vi "AnalogOutput_PanelSim_Global.vi"(0 "menu":T4=enum."get", 5 "AO Channel":T3=enum."Invalid", 9 "Value Set":dbl format="%#.4f", 11 "error in (no error)":errorcluster, 12 "JSON":string) -> (10 "Value get":T1={"type"="AO", "device"="", "name"="", "data"={"<init"=FALSE, "<voltage"=0.0}}, 15 "error out":errorcluster)   [LabVIEW 2019]
doc: "This is used to set and get the last motor output values. This is needed for simulation, since we cannot read these values from the hardware.\n\nThis software is licensed. Open the labview\\readme\\WPI Robotics Library Open Source License.txt file for more information."
uses:
  AO Update Ops.ctl
  AO proto.ctl
  AO Data proto.ctl
  <vilib>/Rock Robotics/WPI/AnalogOutput/WPI_AnalogOutputChannel.ctl
panel:
  out "All Values":T1[](array[typedef])
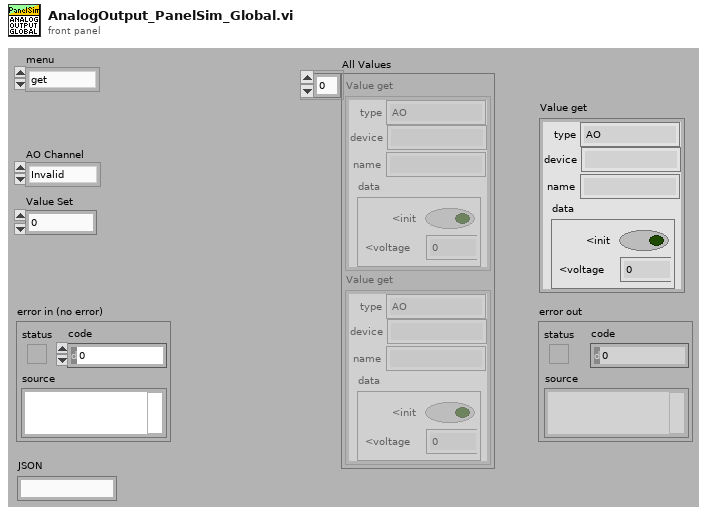
[diagram p1: front panel]
types:
  T1 = typedef "AO proto.ctl" = cluster{"type":string, "device":string, "name":string, "data":T2}
  T2 = typedef "AO Data proto.ctl" = cluster{"<init":bool, "<voltage":dbl}
  T3 = typedef "WPI_AnalogOutputChannel.ctl" = enum8{"AO MXP 0", "AO MXP 1", "Invalid"}
  T4 = typedef "AO Update Ops.ctl" = enum16{"set init", "set value", "JSON update", "set name", "transmit initial", "get", "delete", "reset"}
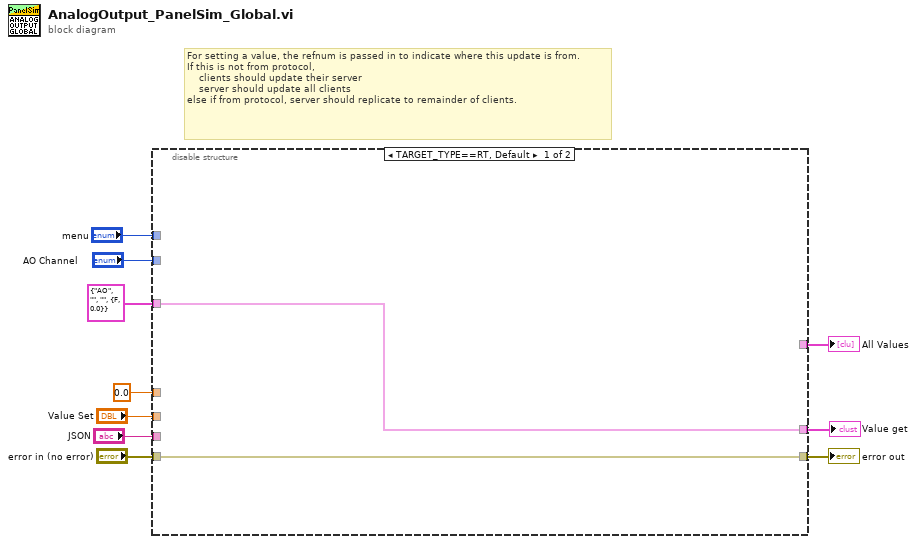
[diagram p0: block diagram]
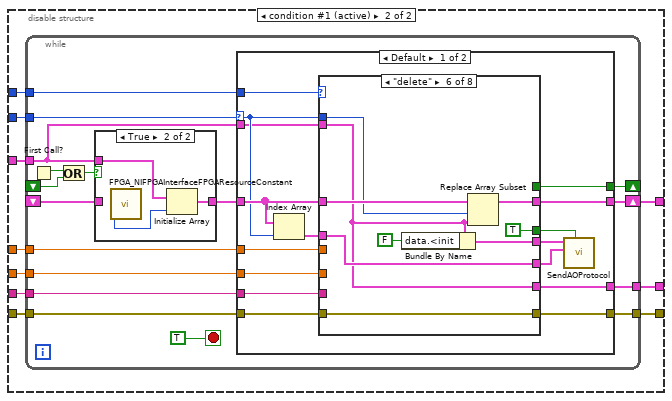
[diagram p2: hidden frame]
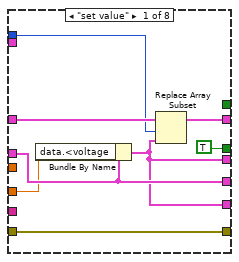
[diagram p3: hidden frame]
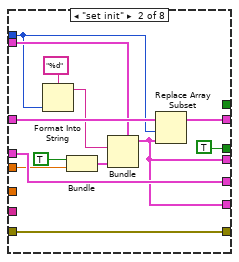
[diagram p4: hidden frame]
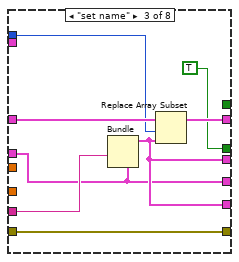
[diagram p5: hidden frame]
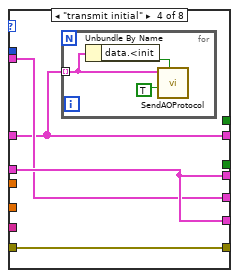
[diagram p6: hidden frame]
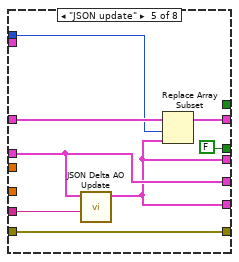
[diagram p7: hidden frame]
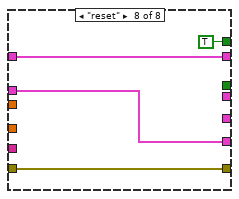
[diagram p9: hidden frame]
diagram:
  # "For setting a value, the refnum is passed in to indicate where this update is from.\nIf this is not from protocol,\n    clients should update their server\n    server should update all clients\nelse if from protocol, server should replicate to remainder of clients."
  n1 = disable-structure shown="TARGET_TYPE==RT, Default" {
    disable-tunnel: "menu" -> [_ w22]
    disable-tunnel: [w12 w21] -> w9
    disable-tunnel: "error in (no error)" -> [w12 w20]
    disable-tunnel: [_ w19] -> w7
    disable-tunnel: 0.0 ("Output") -> [_ w18]
    disable-tunnel: "Value Set" -> [_ w17]
    disable-tunnel: "AO Channel" -> [_ w16]
    disable-tunnel: [w11 w15] -> w3
    disable-tunnel: "JSON" -> [_ w14]
    disable-tunnel: T1 {"type"="AO", "device"="", "name"="", "data"={"<init"=FALSE, "<voltage"=0.0}} ("data") -> [w11 w13]
    frame condition #0 {
    }
    frame condition #1 (active) {
      n2 = while {
        tunnel: w17 -> [w39]
        tunnel: w20 -> [w35]
        shift-right: [w38] -> w19
        shift-left: _ -> [w31]
        tunnel: [w37] -> w15
        tunnel: w22 -> [w36]
        tunnel: [w34] -> w21
        tunnel: w16 -> [w29]
        tunnel: w18 -> [w30]
        tunnel: w14 -> [w28]
        tunnel: w13 -> [w27]
        shift-right: [w23] -> _
        shift-left: _ -> [w24]
        stop <- TRUE stop-if-true
        n3 = First Call?() -> (First Call?: T/F=w25:bool)
        n4 = Or(x=w25, y=w24) -> (x .or. y?=w26:bool)
        n5 = case shown="True" w26 {
          tunnel: [w119 w122] -> w32
          tunnel: w31 -> [w119 _]
          tunnel: w27 -> [_ w120]
          frame False {
          }
          frame True {
            n6 = call <vilib>:"FPGA_NIFPGAInterfaceFPGAResourceConstant.vi"() -> ("NumberOfAOChannels"=w121:u8)  [unwired: 11 out]
            n7 = Initialize Array(w120, w121) -> (w122:T1[])
          }
        }
        n8 = case shown="Default" w29 {
          selector: w29 -> [w47 _]
          tunnel: w39 -> [w55 _]
          tunnel: [w54 w118] -> w38
          tunnel: [w53 w116] -> w37
          tunnel: w36 -> [w52 _]
          tunnel: w35 -> [w51 w117]
          tunnel: [w50 w117] -> w34
          tunnel: w32 -> [w49 w118]
          tunnel: w30 -> [w48 _]
          tunnel: w28 -> [w42 _]
          tunnel: w27 -> [w41 w116]
          tunnel: [w40 _] -> w23
          frame Default {
            n9 = Index Array(array=w49, index=w47) -> (element=w46:T1)
            n10 = case shown="\"delete\"" w52 {
              tunnel: w55 -> [w57 _ _ _ _ _ _ _]
              tunnel: [w63 w76 w84 w85 w99 w107 w111 w115] -> w54
              tunnel: w49 -> [w61 w74 w82 w85 w97 w108 w111 w115]
              tunnel: [w56 w68 w79 w87 w92 w102 w109 w113] -> w53
              tunnel: [w62 w75 w83 w88 w98 w106 w110 w114] -> w50
              tunnel: w51 -> [w62 w75 w83 w88 w98 w106 w110 w114]
              tunnel: w47 -> [w59 w67 w80 _ w95 w103 _ _]
              tunnel: w48 -> [_ w64 _ _ _ _ _ _]
              tunnel: [w56 w68 w79 w87 w92 w101 _ _] -> w44
              tunnel: [w58 w72 w77 w86 w93 w104 _ _] -> w45
              tunnel: [TRUE TRUE TRUE _ FALSE TRUE _ _] -> w43
              tunnel: w46 -> [w58 w72 w77 w87 w93 w104 w109 w113]
              tunnel: w42 -> [_ _ w78 _ w94 _ _ _]
              tunnel: w41 -> [_ w71 _ w86 _ w102 _ _]
              tunnel: [_ _ _ _ _ _ _ TRUE] -> w40
              frame "set value" {
                n11 = Bundle By Name(cluster=w58, "data.<voltage"=w57) -> (w56:T1)
                n12 = Replace Array Subset(array=w61, new element=w56, index=w59) -> (w63:T1[])
              }
              frame "set init" {
                n13 = Format Into String(format string="%d", w67) -> (resulting string=w65:string)  [unwired: 2 in, 1 out]
                n14 = Bundle(TRUE, "Output"=w64) -> (w69:cluster{bool, "Output":dbl})  [unwired: 1 in]
                n15 = Bundle(cluster=w71, "device"=w65, "data"=w69) -> (w68:T1)  [unwired: 2 in]
                n16 = Replace Array Subset(array=w74, new element=w68, index=w67) -> (w76:T1[])
              }
              frame "set name" {
                n17 = Bundle(cluster=w77, "name"=w78) -> (w79:T1)  [unwired: 3 in]
                n18 = Replace Array Subset(array=w82, new element=w79, index=w80) -> (w84:T1[])
              }
              frame "transmit initial" {
                n19 = for {
                  tunnel: w85 -> [w90] mode=indexing
                  n20 = Unbundle By Name(w90) -> ("data.<init"=w89:bool)
                  n21 = call "SendAOProtocol.vi"("Send"=w89, "Initialize"=TRUE, "new"=w90) -> ()  [unwired: 9 in]
                }
              }
              frame "JSON update" {
                n22 = call "JSON Delta AO Update.vi"("Delta JSON"=w94, "input"=w93) -> ("output"=w92:T1)  [unwired: 8 in, 1 out]
                n23 = Replace Array Subset(array=w97, new element=w92, index=w95) -> (w99:T1[])
              }
              frame "delete" {
                n24 = Bundle By Name(cluster=w102, "data.<init"=FALSE) -> (w101:T1)
                n25 = Replace Array Subset(array=w108, new element=w102, index=w103) -> (w107:T1[])
              }
              frame "get" {
              }
              frame "reset" {
              }
            }
            n26 = call "SendAOProtocol.vi"("Send"=w43, "prev"=w45, "new"=w44) -> ()  [unwired: 9 in]
          }
          frame "Invalid" {
            # "Do nothing if \nchannel is Invalid."
          }
        }
      }
    }
  }
  "error out" <- w9
  "All Values" <- w7
  "Value get" <- w3
